vi "dutCyc2.vi"() -> ()   [LabVIEW 2017]
uses:
  <vilib>/myRIO/Instrument Drivers/Onboard IO/DIO/typedefs/DIO Reference.ctl
  <vilib>/myRIO/Common/Instrument Driver Framework/Utilities/typedefs/myRIO Generic Hardware Reference.ctl
  <vilib>/myRIO/Common/Instrument Driver Framework/Utilities/typedefs/Hardware Version Enum.ctl
  <vilib>/myRIO/Common/Instrument Driver Framework/Utilities/typedefs/myRIO v1.0 Reference.ctl
  <vilib>/myRIO/Common/Instrument Driver Framework/Utilities/typedefs/Generic FPGA Reference.ctl
  <vilib>/myRIO/Common/Instrument Driver Framework/myRIO v1.0/DIO/typedefs/DIO Channels List.ctl
  <vilib>/myRIO/Common/Instrument Driver Framework/myRIO v1.0/DIO/typedefs/DIO Channels Enum.ctl
  <vilib>/userdefined/High Color/nirio_resource_hc.ctl
  <vilib>/myRIO/Instrument Drivers/Onboard IO/PWM/typedefs/PWM Reference.ctl
  <vilib>/myRIO/Common/Instrument Driver Framework/myRIO v1.0/PWM/typedefs/PWM Channels Enum.ctl
  <vilib>/myRIO/Instrument Drivers/Onboard IO/PWM/typedefs/PWM Configuration.ctl
  <vilib>/myRIO/Common/Instrument Driver Framework/Utilities/vis/Is FPGA Ref Available.vi
  <vilib>/myRIO/Common/Instrument Driver Framework/myRIO v1.0/DIO/vis/myRIO v1.1 Open DIO.vi
  <vilib>/myRIO/Instrument Drivers/Onboard IO/DIO/vis/Write.vi
  <vilib>/myRIO/Common/Instrument Driver Framework/myRIO v1.0/PWM/vis/myRIO v1.1 Open PWM.vi
  <vilib>/myRIO/Instrument Drivers/Onboard IO/PWM/vis/Set Duty Cycle and Frequency.vi
  <vilib>/myRIO/Common/Instrument Driver Framework/myRIO v1.0/UART/vis/myRIO v1.0 Close UART.vi
  <vilib>/myRIO/Common/Instrument Driver Framework/Utilities/vis/Validate Channels.vi
  <vilib>/myRIO/Common/Instrument Driver Framework/myRIO v1.0/DIO/vis/myRIO v1.0 Reserve DIO.vi
  <vilib>/myRIO/Common/Instrument Driver Framework/myRIO v1.0/PWM/vis/myRIO v1.0 Reserve PWM.vi
  <vilib>/myRIO/Common/Instrument Driver Framework/myRIO v1.0/Resource Manager/vis/myRIO v1.0 Reserve Channel List.vi
  <vilib>/myRIO/Common/Instrument Driver Framework/myRIO v1.0/DIO/vis/myRIO v1.0 Build MUX Configuration DIO.vi
  <vilib>/myRIO/Common/Instrument Driver Framework/myRIO v1.0/PWM/vis/myRIO v1.0 Build MUX Configuration PWM.vi
  <vilib>/myRIO/Common/Instrument Driver Framework/myRIO v1.0/Resource Manager/vis/myRIO v1.0 Reserve Channel.vi
  <vilib>/myRIO/Common/Instrument Driver Framework/myRIO v1.0/Resource Manager/vis/myRIO v1.0 Unreserve Channel.vi
  <vilib>/myRIO/Common/Instrument Driver Framework/myRIO v1.0/Resource Manager/vis/myRIO v1.0 Create Configuration List.vi
  <vilib>/myRIO/Common/Instrument Driver Framework/myRIO v1.0/Resource Manager/vis/myRIO v1.0 Build Mutex Name.vi
  <vilib>/myRIO/Common/Instrument Driver Framework/Utilities/vis/FPGA Ref Manager.vi
  <vilib>/myRIO/Common/Instrument Driver Framework/myRIO v1.0/myRIO v1.0 Reset FPGA.vi
  <vilib>/myRIO/Common/Instrument Driver Framework/myRIO v1.0/IRQ/vis/myRIO v1.0 IRQ Info FGV.vi
  <vilib>/myRIO/Common/Instrument Driver Framework/myRIO v1.0/IRQ/vis/myRIO v1.0 Timer IRQ Info FGV.vi
  <vilib>/myRIO/Common/Instrument Driver Framework/myRIO v1.0/IRQ/vis/myRIO v1.0 ISR Agent.vi
  <vilib>/Utility/VariantDataType/GetNumericInfo.vi
  <vilib>/Utility/error.llb/Error Cluster From Error Code.vi
  <vilib>/myRIO/Common/Instrument Driver Framework/myRIO v1.0/myRIO v1.1 Open.vi
  <vilib>/myRIO/Common/Instrument Driver Framework/Utilities/vis/IO Manager.vi
  <vilib>/myRIO/Common/Instrument Driver Framework/Utilities/vis/Configuration Manager.vi
  <vilib>/myRIO/Common/Instrument Driver Framework/myRIO v1.0/Resource Manager/vis/myRIO v1.0 Configure IO.vi
  <vilib>/myRIO/Common/Instrument Driver Framework/myRIO v1.0/myRIO v1.0 Close.vi
  <vilib>/myRIO/Common/Instrument Driver Framework/myRIO v1.0/DIO/vis/myRIO v1.0 Write DIO.vi
  <vilib>/myRIO/Common/Instrument Driver Framework/myRIO v1.0/PWM/vis/myRIO v1.0 Write PWM.vi
  <vilib>/myRIO/Express VI/Onboard IO/DO/DO Express VI.xnode
  <vilib>/myRIO/Instrument Drivers/Onboard IO/DIO/vis/myRIO DIO Open.xnode
  <vilib>/myRIO/Express VI/Onboard IO/PWM/PWM Express VI.xnode
  <vilib>/myRIO/Instrument Drivers/Onboard IO/PWM/vis/myRIO PWM Open.xnode
  <vilib>/myRIO/Instrument Drivers/Utilities/Utilities.lvlib
  <vilib>/myRIO/Instrument Drivers/Onboard IO/DIO/DIO.lvlib
  <vilib>/myRIO/Instrument Drivers/Onboard IO/PWM/PWM.lvlib
panel:
  in  "Duty cycle":dbl
  out "TestVar":dbl
  in  "Stop Button":bool
  out "error out":errorcluster
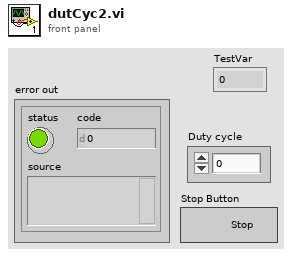
[diagram p1: front panel]
types:
  T1 = typedef "PWM.lvlib/PWM Reference.ctl" = cluster{"myRIO Reference":T2, "PWM Channels Enum":T6, "PWM Configuration":T7}
  T2 = typedef "myRIO Generic Hardware Reference.ctl" = cluster{"myRIO Model":T3, "myRIO Hardware Reference":T4}
  T3 = typedef "Hardware Version Enum.ctl" = enum16{"Unknown", "myRIO-1900", "myRIO-1950", "roboRIO", "NI ELVIS RIO CM"}
  T4 = typedef "myRIO v1.0 Reference.ctl" = cluster{"Generic FPGA Reference":T5, "Allow multiple opens":bool}
  T5 = typedef "Generic FPGA Reference.ctl" = refnum<k20>
  T6 = typedef "PWM Channels Enum.ctl" = enum16{"Not Connected", "C/PWM0", "C/PWM1", "A/PWM0", "A/PWM1", "A/PWM2", "B/PWM0", "B/PWM1", "B/PWM2", "PWM/PWM0", "PWM/PWM1", "PWM/PWM2", "PWM/PWM3", "PWM/PWM4", "PWM/PWM5", "PWM/PWM6", "PWM/PWM7", "PWM/PWM8", "PWM/PWM9"}
  T7 = typedef "PWM.lvlib/PWM Configuration.ctl" = cluster{"Frequency":dbl, "Duty Cycle":dbl}
  T8 = typedef "nirio_resource_hc.ctl" = tag
  T9 = typedef "DIO.lvlib/DIO Reference.ctl" = cluster{"myRIO Reference":T2, "DIO Channels List":T10}
  T10 = typedef "DIO Channels List.ctl" = T11[]
  T11 = typedef "DIO Channels Enum.ctl" = enum16{"Not Connected", "C/DIO0", "C/DIO1", "C/DIO2", "C/DIO3", "C/DIO4", "C/DIO5", "C/DIO6", "C/DIO7", "A/DIO0", "A/DIO1", "A/DIO2", "A/DIO3", "A/DIO4", "A/DIO5", "A/DIO6", "A/DIO7", "A/DIO8", "A/DIO9", "A/DIO10", "A/DIO11", "A/DIO12", "A/DIO13", "A/DIO14", "A/DIO15", "B/DIO0", "B/DIO1", "B/DIO2", "B/DIO3", "B/DIO4", "B/DIO5", "B/DIO6", "B/DIO7", "B/DIO8", "B/DIO9", "B/DIO10", "B/DIO11", "B/DIO12", "B/DIO13", "B/DIO14", "B/DIO15", "LED0", "LED1", "LED2", "LED3", "Button0", "DIO/DIO0", "DIO/DIO1", "DIO/DIO2", "DIO/DIO3", "DIO/DIO4", "DIO/DIO5", "DIO/DIO6", "DIO/DIO7", "DIO/DIO8", "DIO/DIO9", "SPI/CS0", "SPI/CS1", "SPI/CS2", "SPI/CS3", "LED RADIO (Green)", "LED RADIO (Red)", "LED COMM (Green)", "LED COMM (Red)", "LED MODE (Green)", "LED MODE (Red)"}
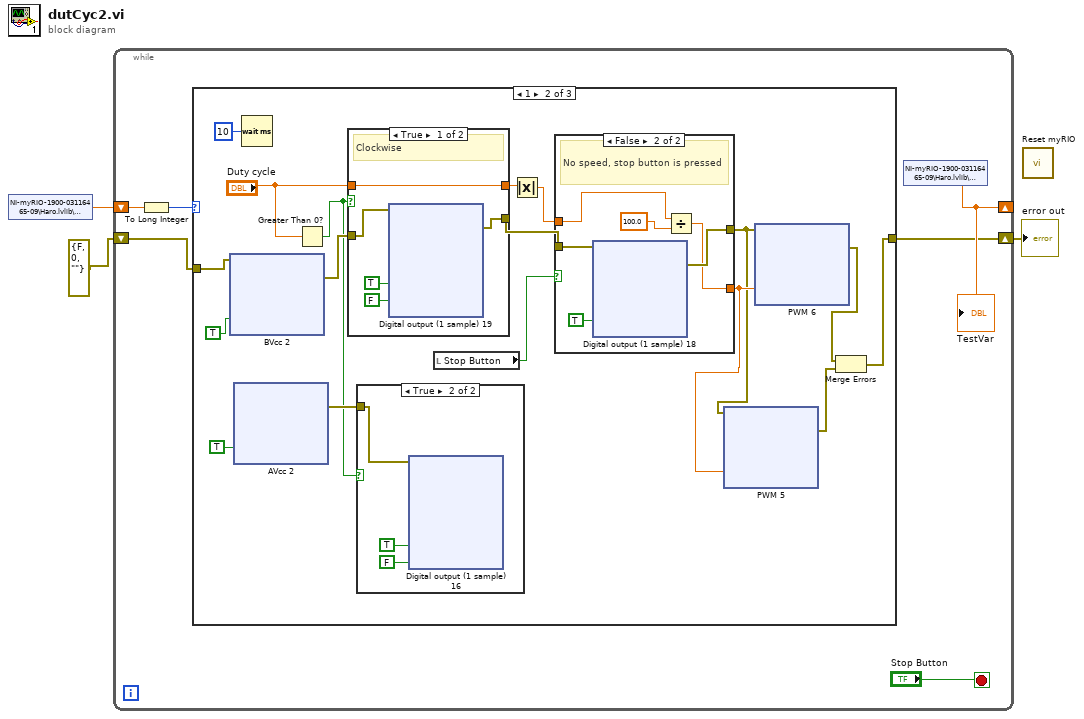
[diagram p0: block diagram]
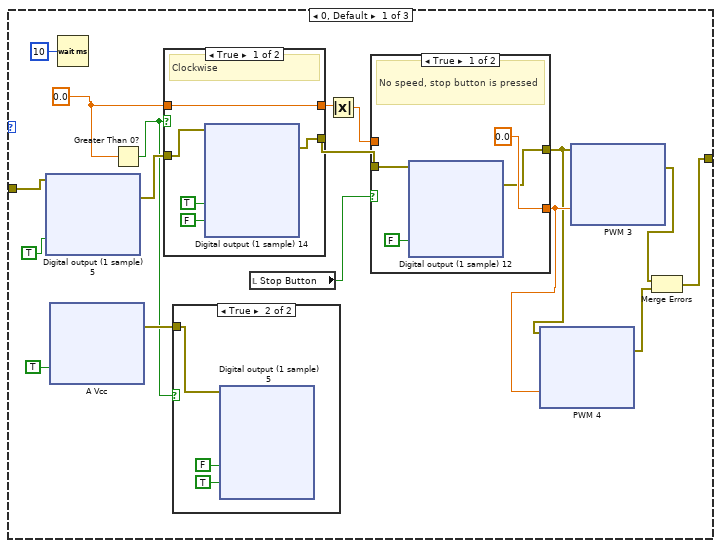
[diagram p2: hidden frame]
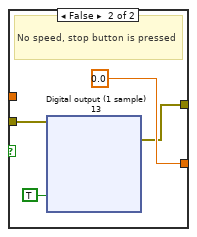
[diagram p4: hidden frame]
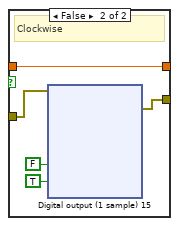
[diagram p5: hidden frame]
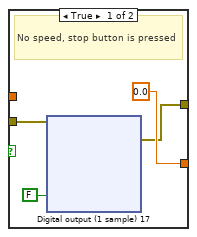
[diagram p7: hidden frame]
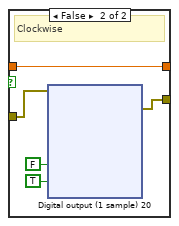
[diagram p8: hidden frame]
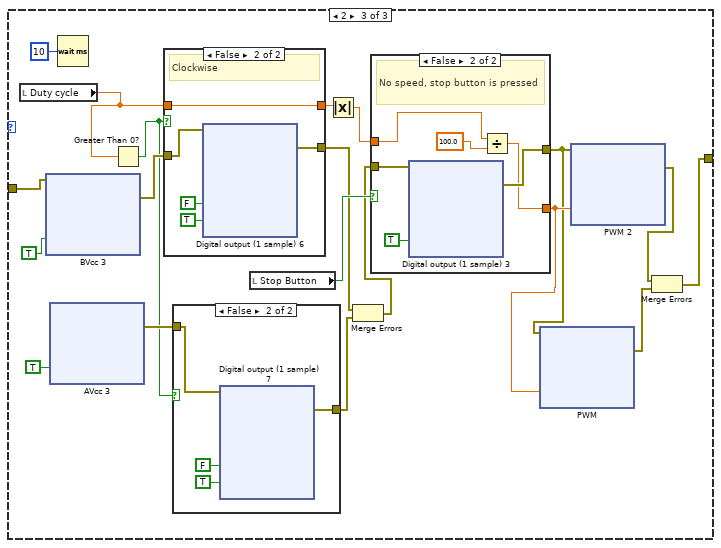
[diagram p9: hidden frame]
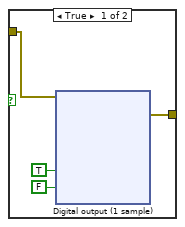
[diagram p10: hidden frame]
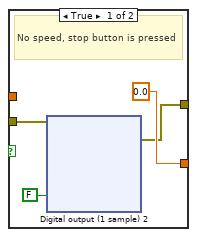
[diagram p11: hidden frame]
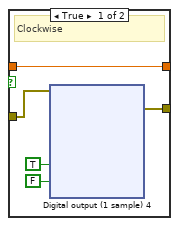
[diagram p12: hidden frame]
diagram:
  n1 = shared-variable "NI-myRIO-1900-03116465-09\\Haro.lvlib\\TestVar"() -> (w3:dbl)  [unwired: 1 in, 1 out]
  n2 = while {
    shift-right: [w8] -> _
    shift-left: w3 -> [w7]
    shift-right: [w5] -> w2
    shift-left: errorcluster {"status"=FALSE, "code"=0, "source"=""} ("error constant") -> [w4]
    stop <- "Stop Button" stop-if-true
    n3 = To Long Integer(number=w7) -> (32bit integer=w6:i32)
    n4 = case shown="1" w6 {
      tunnel: [w11 w368 w729] -> w5
      tunnel: w4 -> [w19 w376 w737]
      frame 0, Default {
        w20 = 0.0 ("Duty Cycle")
        n5 = xnode "Digital output (1 sample) 5"("BVcc (B/DIO3 (Pin 17))"=TRUE ("Vcc (A/DIO3 (Pin 17))"), "error in (no error)"=w19) -> ("error out"=w23:errorcluster)
        n6 = xnode "A Vcc"("AVcc (A/DIO3 (Pin 17))"=TRUE) -> ("error out"=w18:errorcluster)  [unwired: 1 in]
        n7 = Wait (ms)(milliseconds to wait=u32 10) -> ()  [unwired: 1 out]
        n8 = Greater Than 0?(x=w20) -> (x > 0?=w17:bool)
        n9 = case shown="True" w17 {
          tunnel: w20 -> [w288 w329]
          tunnel: [w288 w329] -> w25
          tunnel: w23 -> [w286 w327]
          tunnel: [w287 w328] -> w22
          frame True {
            # "Clockwise"
            n10 = xnode "Digital output (1 sample) 14"("Bin2 (B/DIO0 (Pin 11))"=TRUE ("Ain2 (A/DIO0 (Pin 11))"), "Bin1 (B/DIO1 (Pin 13))"=FALSE ("Ain1 (A/DIO1 (Pin 13))"), "error in (no error)"=w286) -> ("error out"=w287:errorcluster)
          }
          frame False {
            # "Clockwise"
            n11 = xnode "Digital output (1 sample) 15"("Bin2 (B/DIO0 (Pin 11))"=FALSE ("Ain2 (A/DIO0 (Pin 11))"), "Bin1 (B/DIO1 (Pin 13))"=TRUE ("Ain1 (A/DIO1 (Pin 13))"), "error in (no error)"=w327) -> ("error out"=w328:errorcluster)
          }
        }
        n12 = case shown="True" w17 {
          tunnel: w18 -> [_ w62]
          frame False {
          }
          frame True {
            n13 = xnode "Digital output (1 sample) 5"("Ain2 (A/DIO0 (Pin 11))"=FALSE, "Ain1 (A/DIO1 (Pin 13))"=TRUE, "error in (no error)"=w62) -> ()  [unwired: 1 out]
          }
        }
        n14 = local read "Stop Button"() -> (w21:bool)
        n15 = Absolute Value(x=w25) -> (abs(x)=w24:dbl)
        n16 = case shown="True" w21 {
          tunnel: w24 -> [_ _]
          tunnel: [0.0 ("Duty Cycle") 0.0 ("Duty Cycle")] -> w14
          tunnel: [w208 w247] -> w10
          tunnel: w22 -> [w207 w246]
          frame True {
            # "No speed, stop button is pressed"
            n17 = xnode "Digital output (1 sample) 12"("stby (B/DIO2 (Pin 15))"=FALSE ("stby (A/DIO2 (Pin 15))"), "error in (no error)"=w207) -> ("error out"=w208:errorcluster)
          }
          frame False {
            # "No speed, stop button is pressed"
            n18 = xnode "Digital output (1 sample) 13"("Bstby (B/DIO2 (Pin 15))"=TRUE ("stby (A/DIO2 (Pin 15))"), "error in (no error)"=w246) -> ("error out"=w247:errorcluster)
          }
        }
        n19 = xnode "PWM 4"("Duty Cycle"=w14, "error in (no error)"=w10) -> ("error out"=w13:errorcluster)
        n20 = xnode "PWM 3"("Duty Cycle"=w14, "error in (no error)"=w10) -> ("error out"=w12:errorcluster)
        n21 = Merge Errors(w12, w13) -> (w11:errorcluster)
      }
      frame 1 {
        n22 = xnode "BVcc 2"("BVcc (B/DIO3 (Pin 17))"=TRUE ("Vcc (A/DIO3 (Pin 17))"), "error in (no error)"=w376) -> ("error out"=w379:errorcluster)
        n23 = xnode "AVcc 2"("AVcc (A/DIO3 (Pin 17))"=TRUE) -> ("error out"=w375:errorcluster)  [unwired: 1 in]
        n24 = Wait (ms)(milliseconds to wait=u32 10) -> ()  [unwired: 1 out]
        n25 = Greater Than 0?(x="Duty cycle") -> (x > 0?=w374:bool)
        n26 = case shown="True" w374 {
          tunnel: "Duty cycle" -> [w646 w687]
          tunnel: [w646 w687] -> w381
          tunnel: w379 -> [w644 w685]
          tunnel: [w645 w686] -> w378
          frame True {
            # "Clockwise"
            n27 = xnode "Digital output (1 sample) 19"("Bin2 (B/DIO0 (Pin 11))"=TRUE ("Ain2 (A/DIO0 (Pin 11))"), "Bin1 (B/DIO1 (Pin 13))"=FALSE ("Ain1 (A/DIO1 (Pin 13))"), "error in (no error)"=w644) -> ("error out"=w645:errorcluster)
          }
          frame False {
            # "Clockwise"
            n28 = xnode "Digital output (1 sample) 20"("Bin2 (B/DIO0 (Pin 11))"=FALSE ("Ain2 (A/DIO0 (Pin 11))"), "Bin1 (B/DIO1 (Pin 13))"=TRUE ("Ain1 (A/DIO1 (Pin 13))"), "error in (no error)"=w685) -> ("error out"=w686:errorcluster)
          }
        }
        n29 = case shown="True" w374 {
          tunnel: w375 -> [_ w418]
          frame False {
          }
          frame True {
            n30 = xnode "Digital output (1 sample) 16"("Ain2 (A/DIO0 (Pin 11))"=TRUE, "Ain1 (A/DIO1 (Pin 13))"=FALSE, "error in (no error)"=w418) -> ()  [unwired: 1 out]
          }
        }
        n31 = local read "Stop Button"() -> (w377:bool)
        n32 = Absolute Value(x=w381) -> (abs(x)=w380:dbl)
        n33 = case shown="False" w377 {
          tunnel: w380 -> [_ w603]
          tunnel: [0.0 ("Duty Cycle") w601] -> w371
          tunnel: [w564 w606] -> w367
          tunnel: w378 -> [w563 w605]
          frame True {
            # "No speed, stop button is pressed"
            n34 = xnode "Digital output (1 sample) 17"("stby (B/DIO2 (Pin 15))"=FALSE ("stby (A/DIO2 (Pin 15))"), "error in (no error)"=w563) -> ("error out"=w564:errorcluster)
          }
          frame False {
            # "No speed, stop button is pressed"
            n35 = xnode "Digital output (1 sample) 18"("Bstby (B/DIO2 (Pin 15))"=TRUE ("stby (A/DIO2 (Pin 15))"), "error in (no error)"=w605) -> ("error out"=w606:errorcluster)
            n36 = Divide(x=w603, y=100.0 ("Duty Cycle")) -> (x/y=w601:dbl)
          }
        }
        n37 = xnode "PWM 5"("Duty Cycle"=w371, "error in (no error)"=w367) -> ("error out"=w370:errorcluster)
        n38 = xnode "PWM 6"("Duty Cycle"=w371, "error in (no error)"=w367) -> ("error out"=w369:errorcluster)
        n39 = Merge Errors(w369, w370) -> (w368:errorcluster)
      }
      frame 2 {
        n40 = local read "Duty cycle"() -> (w727:dbl)
        n41 = xnode "BVcc 3"("BVcc (B/DIO3 (Pin 17))"=TRUE ("Vcc (A/DIO3 (Pin 17))"), "error in (no error)"=w737) -> ("error out"=w739:errorcluster)
        n42 = xnode "AVcc 3"("AVcc (A/DIO3 (Pin 17))"=TRUE) -> ("error out"=w736:errorcluster)  [unwired: 1 in]
        n43 = Wait (ms)(milliseconds to wait=u32 10) -> ()  [unwired: 1 out]
        n44 = Greater Than 0?(x=w727) -> (x > 0?=w735:bool)
        n45 = case shown="False" w735 {
          tunnel: w727 -> [w1047 w1088]
          tunnel: [w1047 w1088] -> w741
          tunnel: w739 -> [w1046 w1087]
          tunnel: [w1043 w1084] -> w725
          frame True {
            # "Clockwise"
            n46 = xnode "Digital output (1 sample) 4"("Bin2 (B/DIO0 (Pin 11))"=TRUE ("Ain2 (A/DIO0 (Pin 11))"), "Bin1 (B/DIO1 (Pin 13))"=FALSE ("Ain1 (A/DIO1 (Pin 13))"), "error in (no error)"=w1046) -> ("error out"=w1043:errorcluster)
          }
          frame False {
            # "Clockwise"
            n47 = xnode "Digital output (1 sample) 6"("Bin2 (B/DIO0 (Pin 11))"=FALSE ("Ain2 (A/DIO0 (Pin 11))"), "Bin1 (B/DIO1 (Pin 13))"=TRUE ("Ain1 (A/DIO1 (Pin 13))"), "error in (no error)"=w1087) -> ("error out"=w1084:errorcluster)
          }
        }
        n48 = case shown="False" w735 {
          tunnel: w736 -> [w779 w819]
          tunnel: [w778 w818] -> w724
          frame True {
            n49 = xnode "Digital output (1 sample)"("Ain2 (A/DIO0 (Pin 11))"=TRUE, "Ain1 (A/DIO1 (Pin 13))"=FALSE, "error in (no error)"=w779) -> ("error out"=w778:errorcluster)
          }
          frame False {
            n50 = xnode "Digital output (1 sample) 7"("Ain2 (A/DIO0 (Pin 11))"=FALSE, "Ain1 (A/DIO1 (Pin 13))"=TRUE, "error in (no error)"=w819) -> ("error out"=w818:errorcluster)
          }
        }
        n51 = local read "Stop Button"() -> (w738:bool)
        n52 = Absolute Value(x=w741) -> (abs(x)=w740:dbl)
        n53 = Merge Errors(w725, w724) -> (w726:errorcluster)
        n54 = case shown="False" w738 {
          tunnel: w740 -> [_ w1004]
          tunnel: [0.0 ("Duty Cycle") w1002] -> w732
          tunnel: [w965 w1007] -> w728
          tunnel: w726 -> [w964 w1006]
          frame True {
            # "No speed, stop button is pressed"
            n55 = xnode "Digital output (1 sample) 2"("stby (B/DIO2 (Pin 15))"=FALSE ("stby (A/DIO2 (Pin 15))"), "error in (no error)"=w964) -> ("error out"=w965:errorcluster)
          }
          frame False {
            # "No speed, stop button is pressed"
            n56 = xnode "Digital output (1 sample) 3"("Bstby (B/DIO2 (Pin 15))"=TRUE ("stby (A/DIO2 (Pin 15))"), "error in (no error)"=w1006) -> ("error out"=w1007:errorcluster)
            n57 = Divide(x=w1004, y=100.0 ("Duty Cycle")) -> (x/y=w1002:dbl)
          }
        }
        n58 = xnode "PWM"("Duty Cycle"=w732, "error in (no error)"=w728) -> ("error out"=w731:errorcluster)
        n59 = xnode "PWM 2"("Duty Cycle"=w732, "error in (no error)"=w728) -> ("error out"=w730:errorcluster)
        n60 = Merge Errors(w730, w731) -> (w729:errorcluster)
      }
    }
    n61 = shared-variable "NI-myRIO-1900-03116465-09\\Haro.lvlib\\TestVar"() -> (w8:dbl)  [unwired: 1 in, 1 out]
    "TestVar" <- w8
  }
  "error out" <- w2
  n62 = call <vilib>:"Reset myRIO.vi"() -> ()  [unwired: 11 in, 1 out]
